vi "setInstronChannel.vi"(8 "error in (no error)":errorcluster, 10 "Channel":i32, 11 "Protocol_Generic in":refnum<class "Protocol_Generic.lvclass">) -> (0 "error out":errorcluster, 3 "Protocol_Generic out":refnum<class "Protocol_Generic.lvclass">)   [LabVIEW 2011, in "Protocol_Generic.lvclass"]
uses:
  Protocol_Generic.lvclass
  Protocol_Generic.lvclass/Protocol_Generic.ctl
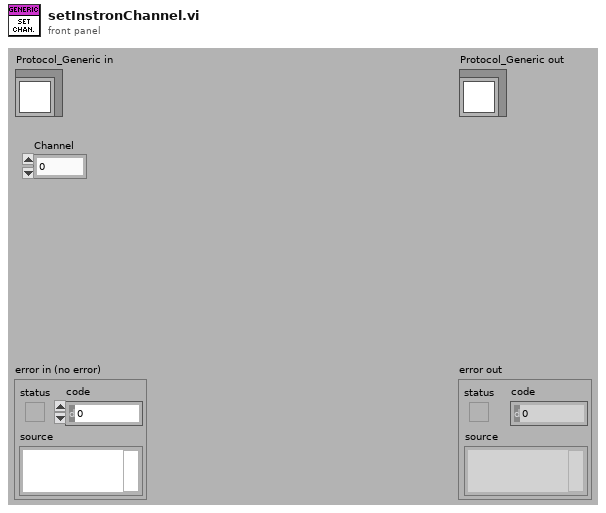
[diagram p1: front panel]
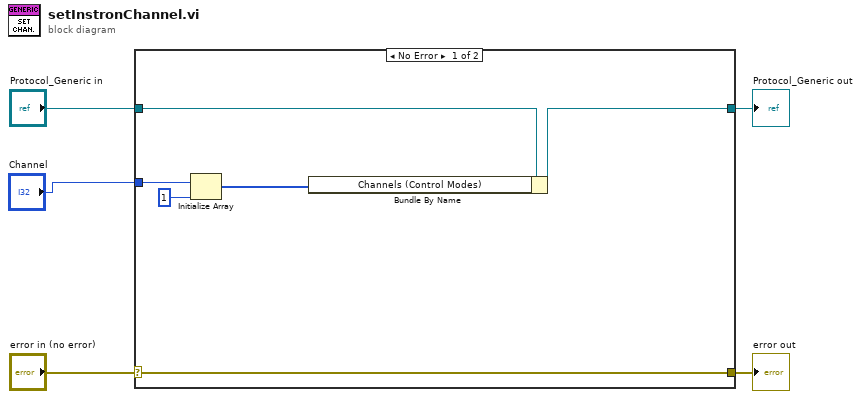
[diagram p0: block diagram]
diagram:
  n1 = case shown="No Error" "error in (no error)" {
    selector: "error in (no error)" -> [w11 w13]
    tunnel: [w11 w13] -> w4
    tunnel: [w6 w12] -> w2
    tunnel: "Protocol_Generic in" -> [w7 w12]
    tunnel: "Channel" -> [w9 _]
    frame No Error {
      n2 = Initialize Array(w9, 1) -> (w8:i32[])
      n3 = Bundle By Name(cluster=w7, "Channels (Control Modes)"=w8) -> (w6:refnum<class "Protocol_Generic.lvclass">)
    }
    frame Error {
    }
  }
  "error out" <- w4
  "Protocol_Generic out" <- w2
